vi "get local pressure from web.vi"() -> (2 "Pressure":dbl[unit], 3 "Pressure (Pa)":dbl)   [LabVIEW 2015]
uses:
  <vilib>/httpClient/LabVIEWHTTPClient.lvlib
panel:
  out "lng":string
  out "lat":string
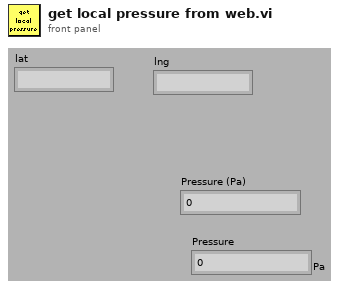
[diagram p1: front panel]
types:
  T1 = typedef "LabVIEWHTTPClient.lvlib/ClientHandle.ctl" = refnum<k1>
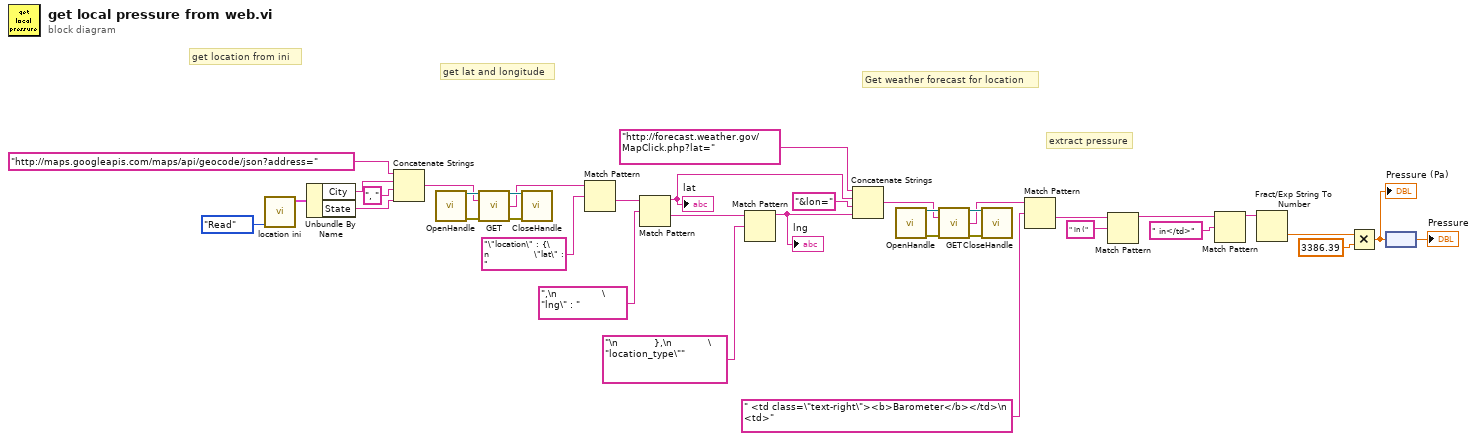
[diagram p0: block diagram]
diagram:
  # "extract pressure"
  # "Get weather forecast for location"
  # "get lat and longitude"
  # "get location from ini"
  n1 = call "location ini.vi"("read/write"=enum16{"Write", "Read"}."Read") -> ("Location Out"=w5:cluster{"City":string, "State":string})  [unwired: 10 in]
  n2 = Unbundle By Name(w5) -> ("City"=w4:string, "State"=w3:string)
  n3 = Concatenate Strings("http://maps.googleapis.com/maps/api/geocode/json?address=" ("URL 2"), w4, ", " ("string"), w3) -> (w27:string)
  n4 = call <vilib>:"OpenHandle.vi"() -> ("client handle out"=w33:T1, "error out"=w32:errorcluster)  [unwired: 14 in]
  n5 = call <vilib>:"GET.vi"("client handle"=w33, "url"=w27, "error in (no error)"=w32) -> ("client handle out"=w31:T1, "body"=w26:string, "error out"=w30:errorcluster)  [unwired: 9 in, 1 out]
  n6 = call <vilib>:"CloseHandle.vi"("client handle"=w31, "error in (no error)"=w30) -> ()  [unwired: 13 in, 1 out]
  n7 = Match Pattern(string=w26, regular expression="\"location\" : {\n               \"lat\" : ") -> (after substring=w23:string)  [unwired: 1 in, 3 out]
  n8 = Match Pattern(string=w23, regular expression=",\n               \"lng\" : ") -> (before substring=w19:string, after substring=w22:string)  [unwired: 1 in, 2 out]
  "lat" <- w19
  n9 = Match Pattern(string=w22, regular expression="\n            },\n            \"location_type\"") -> (before substring=w17:string)  [unwired: 1 in, 3 out]
  "lng" <- w17
  n10 = Concatenate Strings("http://forecast.weather.gov/MapClick.php?lat=", w19, "&lon=" ("string"), w17) -> (w16:string)
  n11 = call <vilib>:"OpenHandle.vi"() -> ("client handle out"=w37:T1, "error out"=w36:errorcluster)  [unwired: 14 in]
  n12 = call <vilib>:"GET.vi"("client handle"=w37, "url"=w16, "error in (no error)"=w36) -> ("client handle out"=w35:T1, "body"=w15:string, "error out"=w34:errorcluster)  [unwired: 9 in, 1 out]
  n13 = call <vilib>:"CloseHandle.vi"("client handle"=w35, "error in (no error)"=w34) -> ()  [unwired: 13 in, 1 out]
  n14 = Match Pattern(string=w15, regular expression=" <td class=\"text-right\"><b>Barometer</b></td>\n            <td>") -> (after substring=w13:string)  [unwired: 1 in, 3 out]
  n15 = Match Pattern(string=w13, regular expression=" in (") -> (before substring=w11:string)  [unwired: 1 in, 3 out]
  n16 = Match Pattern(string=w11, regular expression=" in</td>") -> (before substring=w9:string)  [unwired: 1 in, 3 out]
  n17 = Fract/Exp String To Number(string=w9) -> (number=w8:dbl)  [unwired: 3 in, 1 out]
  n18 = Multiply(x=w8, y=3386.39) -> (x*y=w2:dbl)
  "Pressure (Pa)" <- w2
  n19 = node(w2) -> (→"Pressure":dbl[unit])
